vi "strip VT100.vi"(1 "read buffer":string) -> (0 "result string":string)   [LabVIEW 2018]
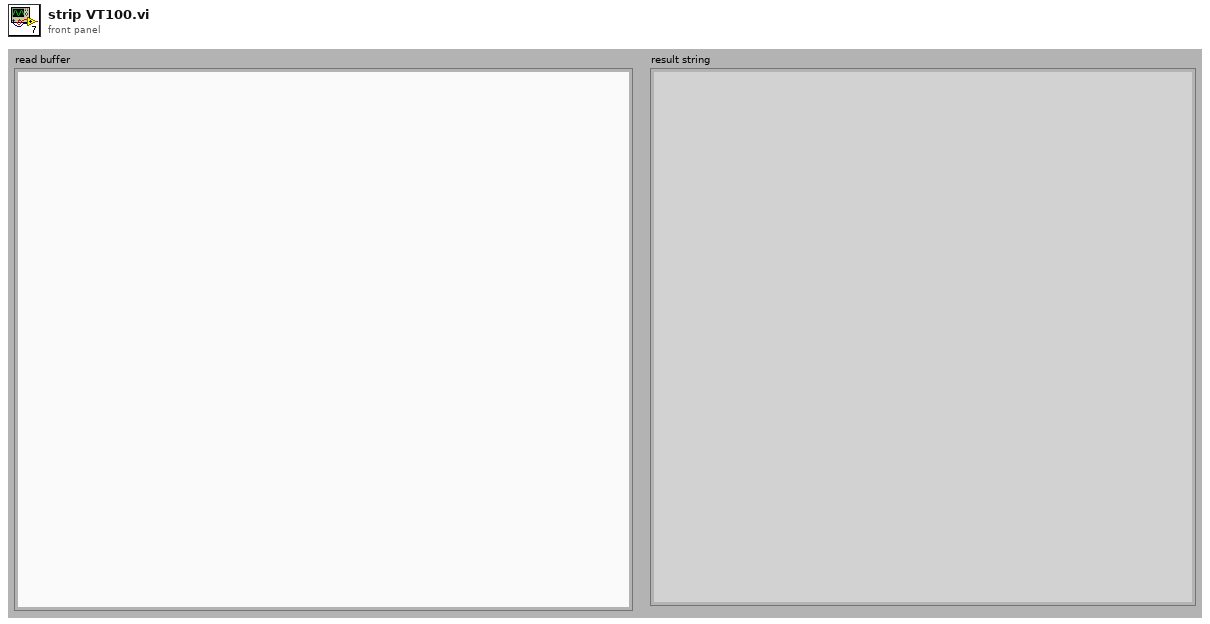
[diagram p1: front panel]
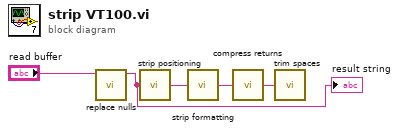
[diagram p0: block diagram]
diagram:
  n1 = call "replace nulls.vi"("read buffer"="read buffer") -> ("result string"=w1:string)  [unwired: 9 in, 1 out]
  "result string" <- w1
  n2 = call "strip positioning.vi"("result string 2"=w1) -> ("result string"=w2:string)
  n3 = call "strip formatting.vi"("result string 2"=w2) -> ("result string"=w3:string)
  n4 = call "compress returns.vi"("result string 2"=w3) -> ("result string"=w4:string)
  n5 = call "trim spaces.vi"("multi-line string"=w4) -> ()  [unwired: 1 out]
